vi "In Higher Series_.vi"(8 "3D sel":T2, 9 "2D sel":T2, 10 "1D sel":T2, 11 "E-Series Data":T3) -> (3 "In Mid-High":T1)   [LabVIEW 2018]
uses:
  E-Series Reader/series data--cluster.ctl
  digit--enum.ctl
  In mid-high series--cluster.ctl
  E-Series Reader/E-Series Reader.lvlib
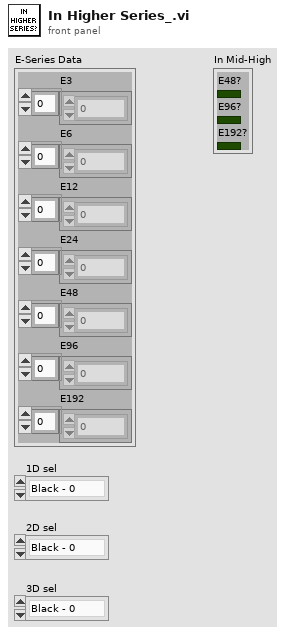
[diagram p1: front panel]
types:
  T1 = typedef "In mid-high series--cluster.ctl" = cluster{"E48?":bool, "E96?":bool, "E192?":bool}
  T2 = typedef "digit--enum.ctl" = enum16{"Black - 0", "Brown - 1", "Red - 2", "Orange - 3", "Yellow - 4", "Green - 5", "Blue - 6", "Violet - 7", "Grey - 8", "White - 9"}
  T3 = typedef "E-Series Reader.lvlib/series data--cluster.ctl" = cluster{"E3":u16[], "E6":u16[], "E12":u16[], "E24":u16[], "E48":u16[], "E96":u16[], "E192":u16[]}
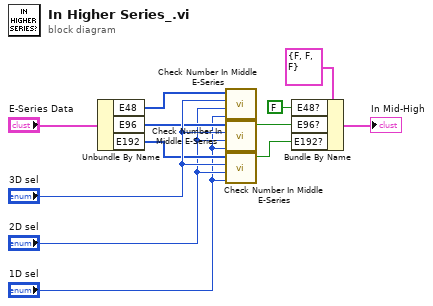
[diagram p0: block diagram]
diagram:
  n1 = Unbundle By Name("E-Series Data") -> ("E48"=w10:u16[], "E96"=w9:u16[], "E192"=w8:u16[])
  n2 = call "Check Number In Middle E-Series.vi"("1D sel"="1D sel", "2D sel"="2D sel", "3D sel"="3D sel", "E Serie"=w10) -> ()  [unwired: 7 in, 1 out]
  n3 = call "Check Number In Middle E-Series.vi"("1D sel"="1D sel", "2D sel"="2D sel", "3D sel"="3D sel", "E Serie"=w9) -> ("In Serie?"=w4:bool)  [unwired: 7 in]
  n4 = call "Check Number In Middle E-Series.vi"("1D sel"="1D sel", "2D sel"="2D sel", "3D sel"="3D sel", "E Serie"=w8) -> ("In Serie?"=w3:bool)  [unwired: 7 in]
  n5 = Bundle By Name(cluster=T1 {"E48?"=FALSE, "E96?"=FALSE, "E192?"=FALSE} ("In Lower"), "E48?"=FALSE, "E96?"=w4, "E192?"=w3) -> (→"In Mid-High":T1)
